vi "esdaq_analogRead.vi"(3 "esdaqErrorInp":errorcluster, 4 "Channel":u8, 5 "esdaqPortInp":refnum<visa-resource-name>) -> (0 "esdaqErrorOut":errorcluster, 1 "value":i32, 2 "esdaqPortOut":refnum<visa-resource-name>)   [LabVIEW 2019]
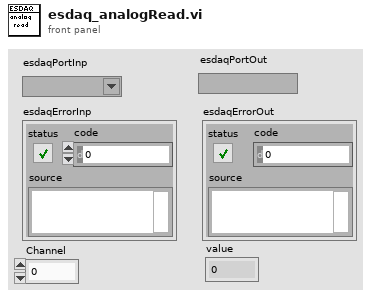
[diagram p1: front panel]
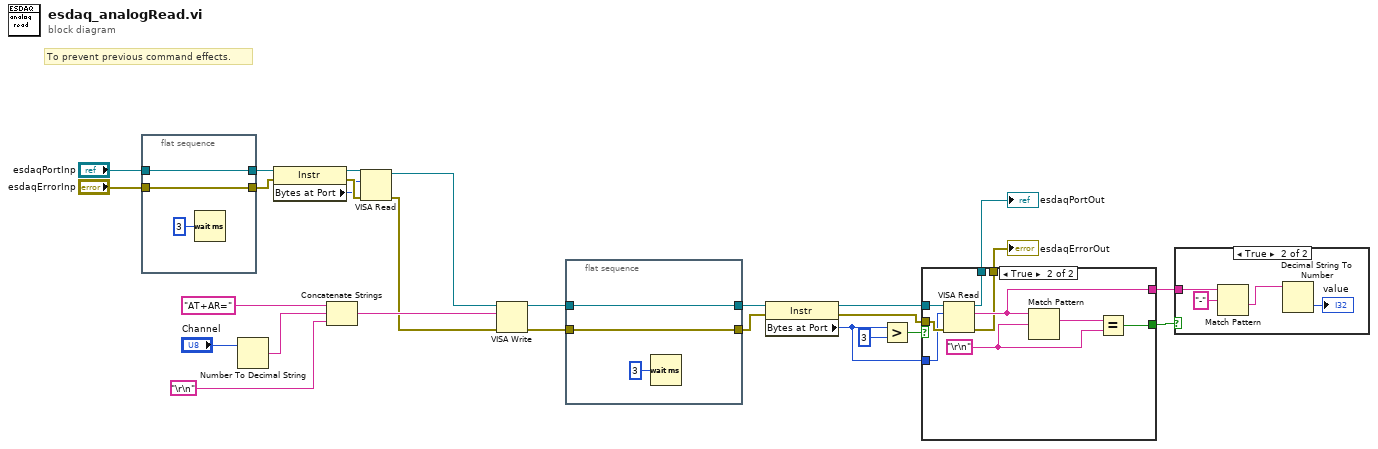
[diagram p0: block diagram]
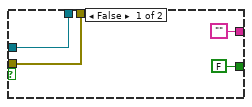
[diagram p3: hidden frame]
diagram:
  # "To prevent previous command effects."
  n1 = flat-sequence {
    tunnel: "esdaqPortInp" -> [w30]
    tunnel: [w30] -> w5
    tunnel: [w29] -> w4
    tunnel: "esdaqErrorInp" -> [w29]
    frame #0 {
      n2 = Wait (ms)(milliseconds to wait=u32 3) -> ()  [unwired: 1 out]
    }
  }
  n3 = Number To Decimal String(number="Channel") -> (decimal integer string=w25:string)  [unwired: 1 in]
  n4 = property class="Instr"(reference=w5, error in=w4) -> (reference out=w10:refnum<visa-resource-name>, error out=w11:errorcluster, "Bytes at Port"=w7:u32)
  n5 = Concatenate Strings("AT+AR=", w25, "\r\n") -> (w24:string)
  n6 = VISA Read(VISA resource name=w10, byte count=w7, error in (no error)=w11) -> (VISA resource name out=w9:refnum<visa-resource-name>, error out=w8:errorcluster)  [unwired: 2 out]
  n7 = VISA Write(VISA resource name=w9, write buffer=w24, error in (no error)=w8) -> (VISA resource name out=w22:refnum<visa-resource-name>, error out=w21:errorcluster)  [unwired: 1 out]
  n8 = flat-sequence {
    tunnel: [w32] -> w20
    tunnel: w22 -> [w32]
    tunnel: [w31] -> w19
    tunnel: w21 -> [w31]
    frame #0 {
      n9 = Wait (ms)(milliseconds to wait=u32 3) -> ()  [unwired: 1 out]
    }
  }
  n10 = property class="Instr"(reference=w20, error in=w19) -> (reference out=w16:refnum<visa-resource-name>, error out=w15:errorcluster, "Bytes at Port"=w14:u32)
  n11 = Greater?(x=w14, y=u32 3) -> (0:w17:bool)
  n12 = case shown="True" w17 {
    tunnel: w16 -> [w35 w46]
    tunnel: w15 -> [w34 w45]
    tunnel: w14 -> [_ w44]
    tunnel: [FALSE w41] -> w13
    tunnel: ["" w40] -> w12
    tunnel: [w35 w39] -> w2
    tunnel: [w34 w38] -> w1
    frame False {
    }
    frame True {
      w42 = "\r\n"
      n13 = VISA Read(VISA resource name=w46, byte count=w44, error in (no error)=w45) -> (VISA resource name out=w39:refnum<visa-resource-name>, read buffer=w40:string, error out=w38:errorcluster)  [unwired: 1 out]
      n14 = Match Pattern(string=w40, regular expression=w42) -> (match substring=w43:string)  [unwired: 1 in, 3 out]
      n15 = Equal?(x=w43, y=w42) -> (x = y?=w41:bool)
    }
  }
  "esdaqPortOut" <- w2
  "esdaqErrorOut" <- w1
  n16 = case shown="True" w13 {
    tunnel: w12 -> [_ w50]
    frame False {
    }
    frame True {
      n17 = Match Pattern(string=w50, regular expression="-") -> (after substring=w48:string)  [unwired: 1 in, 3 out]
      n18 = Decimal String To Number(string=w48) -> (number=→"value":i32)  [unwired: 2 in, 1 out]
    }
  }
